vi "Stop Core.vi"(10 "final error code":i32, 11 "BNT_SLTagMonitor in":refnum<class "BNT_SLTagMonitor.lvclass">) -> (3 "BNT_SLTagMonitor out":refnum<class "BNT_SLTagMonitor.lvclass">)   [LabVIEW 2019, in "BNT_SLTagMonitor.lvlib" / "BNT_SLTagMonitor.lvclass"]
doc: "(<B>Filename</B>: Actor Framework.lvlib:Actor.lvclass:Stop Core.vi)\n\nDefines what the actor does before it stops. Use the <B>final error code</B> input to determine whether the actor shut down in response to an error.\n\nBy default, this method does nothing. A descendant class may override it to define behavior, such as shutting down any processes the actor initiated in its override of the Actor Core method."
uses:
  BNT_SLTagMonitor.lvclass
  CSPP_Core/Actors/CSPP_PVMonitor/CSPP_PVMonitor.lvclass
  <vilib>/event_ctls.llb/usereventprio.ctl
  <vilib>/Skyline/Tag/Wrapper/Wrapper_class/NI Skyline Tag.lvclass
  <vilib>/Skyline/Tag/Wrapper/Wrapper_class/Close Tag (Single).vi
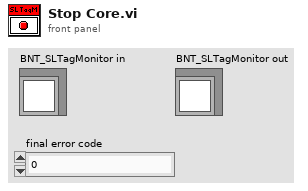
[diagram p1: front panel]
types:
  T1 = typedef "usereventprio.ctl" = enum32{"high priority", "normal priority"}
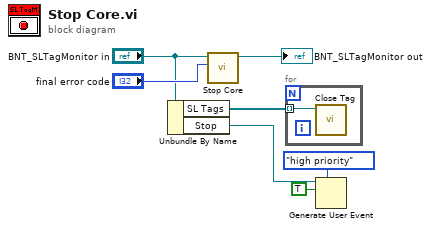
[diagram p0: block diagram]
diagram:
  n1 = Unbundle By Name("BNT_SLTagMonitor in") -> ("SL Tags"=w4:refnum<class "NI Skyline Tag.lvclass">[], "Stop"=w3:refnum<user-event>)
  n2 = call-parent "Stop Core.vi"("final error code"="final error code", "CSPP_BaseActor in"="BNT_SLTagMonitor in") -> ("CSPP_BaseActor out"=→"BNT_SLTagMonitor out":refnum<class "BNT_SLTagMonitor.lvclass">)  [unwired: 9 in]
  n3 = for {
    tunnel: w4 -> [w8] mode=indexing
    n4 = call-poly <vilib>:"Close Tag.vi"("tag"=w8) -> ()  [unwired: 10 in, 1 out]
  }
  n5 = Generate User Event(priority (normal)=usereventprio."high priority", user event=w3, event data cluster=TRUE ("event data")) -> ()  [unwired: 1 in, 2 out]
